vi "DP-Averager (with rejection).vi"(0 "DataAcq":T1, 11 "error in":errorcluster, 12 "Abort":refnum<vi>) -> (6 "Ave Wave":dbl[](graph), 8 "Averaged Spectrum (Vrms)":dbl[](array[numeric]), 14 "waveform cluster":cluster{i32, "dx":dbl, "Array":dbl[]}, 15 "error out":errorcluster)   [LabVIEW 2020]
uses:
  Utility VIs/Math VIs/Linear to dB (array).vi
  Typedefs/DP-DataAcq.ctl
panel:
  out "# Spectra":i32
  out "# Waves":i32
  out "Spectrum":cluster{i32, "dx":dbl, "Array":dbl[]}(graph)
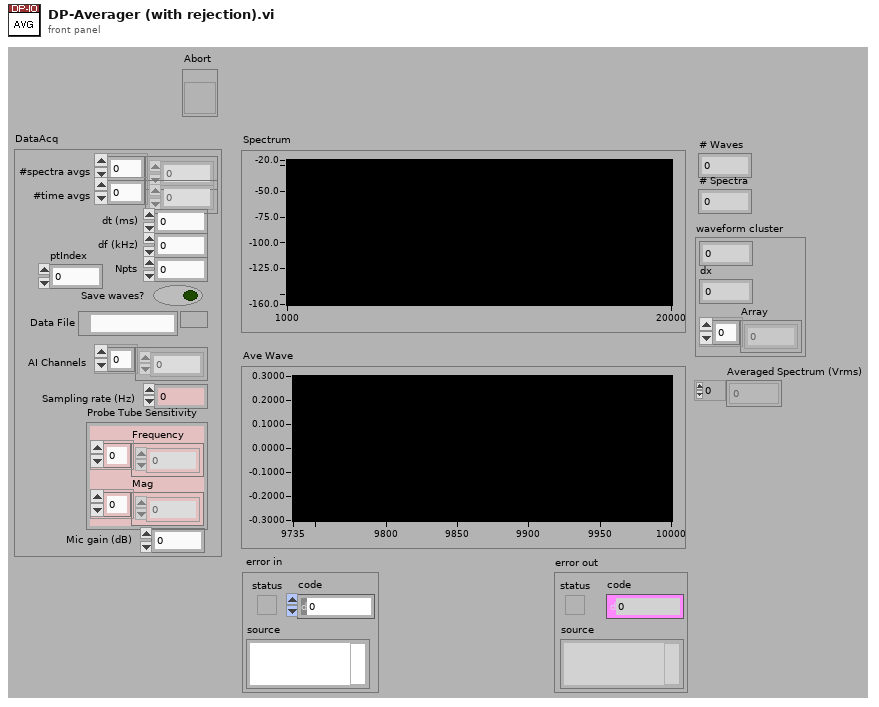
[diagram p1: front panel]
types:
  T1 = typedef "DP-DataAcq.ctl" = cluster{"#spectra avgs":i32[], "#time avgs":i32[], "dt (ms)":dbl, "df (kHz)":dbl, "Npts":i32, "Save waves?":bool, "Data File":path, "AI Channels":u16[], "Sampling rate (Hz)":dbl, "Probe Tube Sensitivity":cluster{"Frequency":dbl[], "Mag":dbl[]}, "Mic gain (dB)":dbl, "ptIndex":i32}
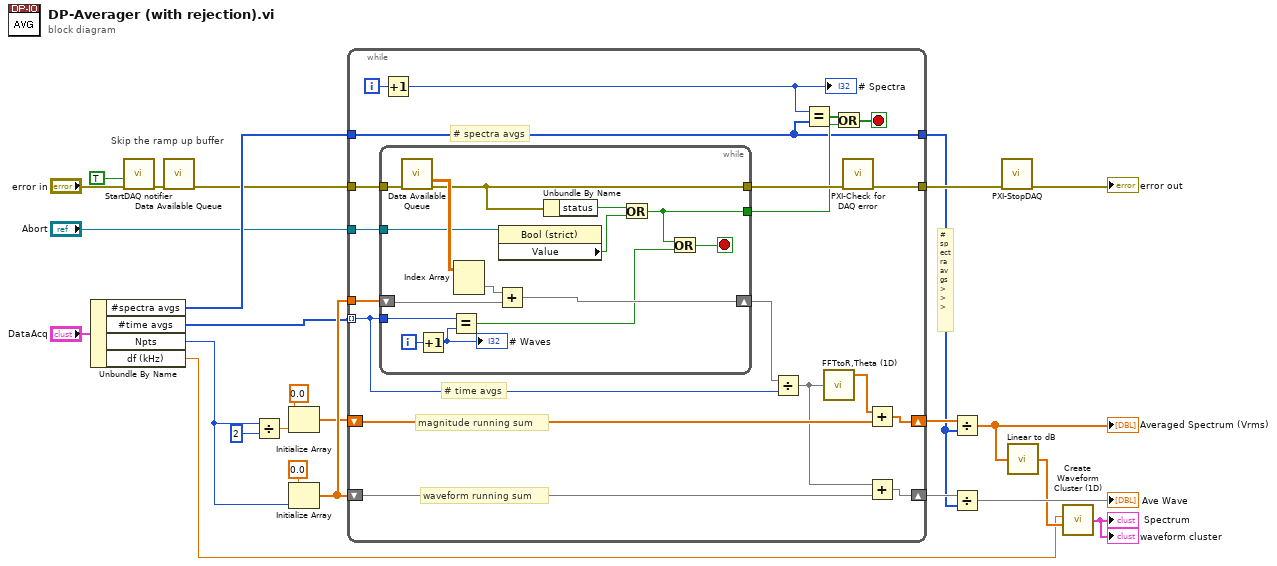
[diagram p0: block diagram]
diagram:
  # "Skip the ramp up buffer"
  # "# spectra avgs>>>"
  n1 = Unbundle By Name("DataAcq") -> ("#spectra avgs"=w11:i32[], "#time avgs"=w10:i32[], "Npts"=w9:i32, "df (kHz)"=w8:dbl)
  n2 = call "StartDAQ notifier.vi"("error in (no error)"="error in", "wait for DAQ? (F)"=TRUE) -> ("error out"=w3:errorcluster)  [unwired: 5 in]
  n3 = call "Data Available Queue.vi"("error in (no error)"=w3) -> ("error out"=w4:errorcluster)  [unwired: 10 in, 4 out]
  n4 = Divide(x=w9, y=2) -> (x/y=w16:dbl)
  n5 = Initialize Array(0.0, w16) -> (w18:dbl[])
  n6 = Initialize Array(0.0, w9) -> (w20:dbl[])
  n7 = while {
    tunnel: w10 -> [w36] mode=indexing
    shift-right: [w43] -> w25
    shift-left: w18 -> [w44]
    shift-right: [w41] -> w23
    shift-left: w20 -> [w42]
    tunnel: w20 -> [w38]
    tunnel: [w29] -> w15
    tunnel: w11 -> [w29]
    tunnel: w4 -> [w40]
    tunnel: [w27] -> w21
    tunnel: "Abort" -> [w26]
    i -> [w35]
    stop <- w31 stop-if-true
    # "# spectra avgs"
    # "# time avgs"
    # "waveform running sum"
    # "magnitude running sum"
    n8 = while {
      shift-right: [w56] -> w37
      shift-left: w38 -> [w57]
      tunnel: w36 -> [w55]
      tunnel: [w48] -> w32
      tunnel: w40 -> [w58]
      tunnel: [w47] -> w39
      tunnel: w26 -> [w46]
      i -> [w54]
      stop <- w50 stop-if-true
      n9 = call "Data Available Queue.vi"("error in (no error)"=w58) -> ("AI Waveforms"=w59:dbl[][], "error out"=w47:errorcluster)  [unwired: 10 in, 3 out]
      n10 = Increment(x=w54) -> (x+1=w53:i32)
      "# Waves" <- w53
      n11 = Equal?(x=w55, y=w53) -> (x = y?=w49:bool)
      n12 = Index Array(array=w59) -> (element=w52:dbl[])  [unwired: 2 in]
      n13 = Add(x=w52, y=w57) -> (x+y=w56:dbl[])
      n14 = property class="Bool (strict)"(reference=w46) -> ("Value"=w45:bool)  [unwired: 1 in, 2 out]
      n15 = Unbundle By Name(w47) -> ("status"=w51:bool)
      n16 = Or(x=w51, y=w45) -> (x .or. y?=w48:bool)
      n17 = Or(x=w48, y=w49) -> (x .or. y?=w50:bool)
    }
    n18 = Increment(x=w35) -> (x+1=w28:i32)
    "# Spectra" <- w28
    n19 = Divide(x=w37, y=w36) -> (x/y=w33:dbl[])
    n20 = Equal?(x=w28, y=w29) -> (x = y?=w30:bool[])
    n21 = call "FFTtoR,Theta (1D).VI"("X"=w33) -> ("+Freq. Mag of FFT"=w34:dbl[])  [unwired: 1 in, 1 out]
    n22 = Or(x=w30, y=w32) -> (x .or. y?=w31:bool[])
    n23 = call "PXI-Check for DAQ error.vi"("error in (no error)"=w39) -> ("error out"=w27:errorcluster)  [unwired: 14 in]
    n24 = Add(x=w34, y=w44) -> (x+y=w43:dbl[])
    n25 = Add(x=w33, y=w42) -> (x+y=w41:dbl[])
  }
  n26 = Divide(x=w25, y=w15) -> (x/y=w14:dbl[])
  "Averaged Spectrum (Vrms)" <- w14
  n27 = Divide(x=w23, y=w15) -> (x/y=→"Ave Wave":dbl[])
  n28 = call "PXI-StopDAQ.vi"("error in (no error)"=w21) -> ("error out"=→"error out":errorcluster)  [unwired: 6 in]
  n29 = call-poly "Linear to dB.vi"("linear"=w14) -> ("dB"=w13:dbl[])
  n30 = call "Create Waveform Cluster (1D).vi"("Array"=w13, "dx"=w8) -> ("waveform cluster"=→"Spectrum" →"waveform cluster":cluster{i32, "dx":dbl, "Array":dbl[]})  [unwired: 2 in]
